vi "Test Stop.vi"(11 "Error in":errorcluster) -> (15 "Error out":errorcluster)   [LabVIEW 2020, in "CelsiusToFarenheitTests.lvlib"]
doc: "This VI is to validate the stop button"
uses:
  CelsiusToFarenheitTests.lvlib
  <vilib>/SLL Drona/APIs/Assert/AssertVI/AssertVIExecRunning.vi
  <vilib>/SLL Drona/APIs/Stimulus/ControlValue/SetValueAuto.vi
  <vilib>/SLL Drona/APIs/Assert/AssertVI/AssertVIExecIdle.vi
  <vilib>/SLL Drona/APIs/Stimulus/VI/CloseVI.vi
  <vilib>/Utility/error.llb/Error Cluster From Error Code.vi
  <vilib>/ErrorRing/Error Ring.xnode
  <vilib>/SLL Drona/Drona.lvlib
  <vilib>/addons/_JKI Toolkits/Caraya/classes/Test/Test.lvclass
  <vilib>/Wiresmith Technology/G CLI/CLI Class/CLI.lvclass
  <vilib>/SLL Drona/APIs/Assert/AssertVI/AssertVI.lvlib
  <vilib>/SLL Drona/APIs/Stimulus/VI/VI.lvlib
  <vilib>/SLL Drona/APIs/Stimulus/ControlValue/ControlValue.lvlib
panel:
  # "STOP BUTTON TEST"
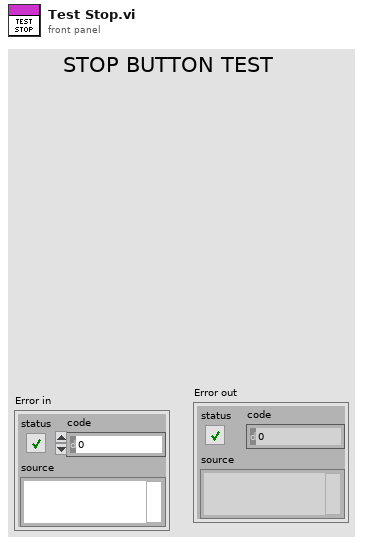
[diagram p1: front panel]
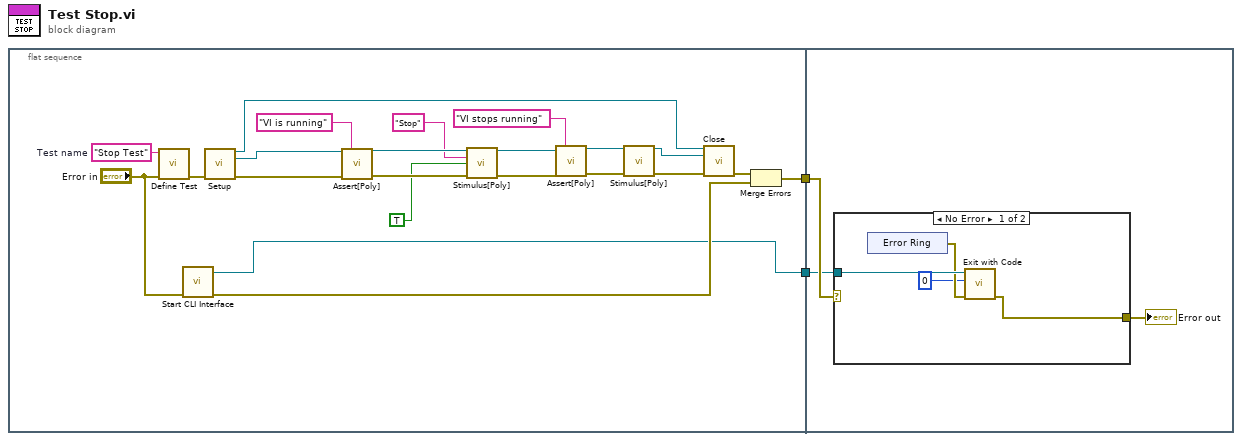
[diagram p0: block diagram]
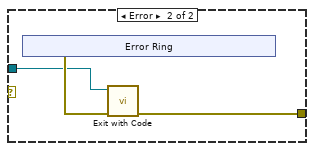
[diagram p2: hidden frame]
diagram:
  n1 = flat-sequence {
    tunnel: [w5] -> w2
    tunnel: [w3] -> w1
    tunnel: w2 -> [w27]
    tunnel: w1 -> [w26]
    frame #0 {
      w23 = "Stop Test"  # Test name
      n2 = call <vilib>:"Define Test.vi"("error in (no error)"="Error in", "Label (VI Title)"=w23) -> ("error out"=w24:errorcluster)  [unwired: 9 in]
      n3 = call <vilib>:"Start CLI Interface.vi"("error in (no error)"="Error in") -> ("error out"=w4:errorcluster, "CLI out"=w3:refnum<class "CLI.lvclass">)  [unwired: 7 in, 2 out]
      n4 = call <vilib>:"Setup.vi"("error in"=w24) -> ("Application Ref"=w22:refnum<vi>, "VI Reference Out"=w19:refnum<vi>, "error out"=w9:errorcluster)  [unwired: 12 in]
      n5 = call-poly <vilib>:"Assert[Poly].vi"("VI Reference In"=w19, "Test Label"="VI is running", "Error In"=w9) -> ("VI Reference Out"=w17:refnum<vi>, "Error Out"=w18:errorcluster)  [unwired: 11 in]
      n6 = call-poly <vilib>:"Stimulus[Poly].vi"("VI Reference In"=w17, "Control Path"="Stop", "Value (Signaling)"=TRUE, "error in"=w18) -> ("VI Reference Out"=w13:refnum<vi>, "error out"=w14:errorcluster)  [unwired: 10 in]
      n7 = call-poly <vilib>:"Assert[Poly].vi"("VI Reference In"=w13, "Test Label"="VI stops running", "Error In"=w14) -> ("VI Reference Out"=w10:refnum<vi>, "Error Out"=w11:errorcluster)  [unwired: 11 in]
      n8 = call-poly <vilib>:"Stimulus[Poly].vi"("VI Reference In"=w10, "error in"=w11) -> ("VI Reference Out"=w21:refnum<vi>, "error out"=w8:errorcluster)  [unwired: 12 in]
      n9 = call <vilib>:"Close.vi"("Application Ref"=w22, "VI Reference"=w21, "error in"=w8) -> ("error out"=w6:errorcluster)  [unwired: 12 in]
      n10 = Merge Errors(w6, w4) -> (w5:errorcluster)
    }
    frame #1 {
      n11 = case shown="No Error" w27 {
        tunnel: w26 -> [w31 w34]
        tunnel: [w30 w33] -> w25
        frame No Error {
          n12 = xnode "Error Ring"() -> ("error out"=w29:errorcluster)
          n13 = call <vilib>:"Exit with Code.vi"("error in (no error)"=w29, "Exit Code (0)"=0, "CLI in"=w31) -> ("error out"=w30:errorcluster)  [unwired: 8 in]
        }
        frame Error {
          n14 = xnode "Error Ring"() -> ("error out"=w35:errorcluster)
          n15 = call <vilib>:"Exit with Code.vi"("error in (no error)"=w35, "CLI in"=w34) -> ("error out"=w33:errorcluster)  [unwired: 9 in]
        }
      }
      "Error out" <- w25
    }
  }
